vi "Protected Channel.vi"(8 "error in (no error)":errorcluster, 11 "Node Ptr":T1 format="%.0x") -> (0 "error out":errorcluster)   [LabVIEW 2015, in "Fuel Injection Addon System Explorer.lvlib"]
uses:
  Fuel Injection Addon System Explorer.lvlib
  <vilib>/NI Veristand/Custom Device API/Custom Device Item Ref.ctl
  <vilib>/NI Veristand/Custom Device API/Custom Device Channel Type.ctl
  <vilib>/NI Veristand/Custom Device API/Custom Device API.lvlib
panel:
  out "Original Name":string
  in  "Default Value":dbl
  out "Units":string
  in  "Header":cluster{"Section Name":string}={"Section Name"="Custom Device Item Settings"}
  in  "Description":string
  in  "Name":string
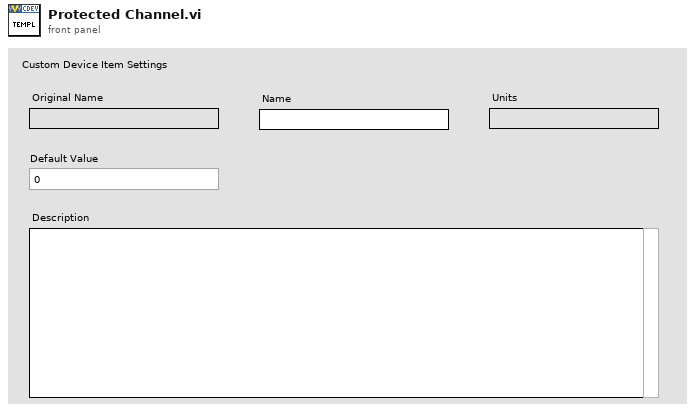
[diagram p1: front panel]
types:
  T1 = typedef "Custom Device API.lvlib/Custom Device Item Ref.ctl" = u64
  T2 = typedef "Custom Device API.lvlib/Custom Device Channel Type.ctl" = enum16{"Input", "Output"}
  T3 = typedef "Custom Device API.lvlib/Custom Device Item Info.ctl" = cluster{"Name":string, "Is Channel":bool, "GUID":string, "Is Waveform":bool}
  T4 = typedef "Custom Device API.lvlib/Custom Device Waveform.ctl" = cluster{"Data Type":T5, "Units":string}
  T5 = typedef "Custom Device API.lvlib/Custom Device Waveform DataType.ctl" = enum16{"Double", "Complex Double"}
  T6 = typedef "Custom Device API.lvlib/Custom Device Channel.ctl" = cluster{"Type":T2, "Units":string, "Default Value":dbl, "Faultable":bool, "Scalable":bool}
  T7 = typedef "Custom Device API.lvlib/Custom Device Commands.ctl" = enum16{"Default", "Item renamed", "Shutdown", "Dynamic button pressed"}
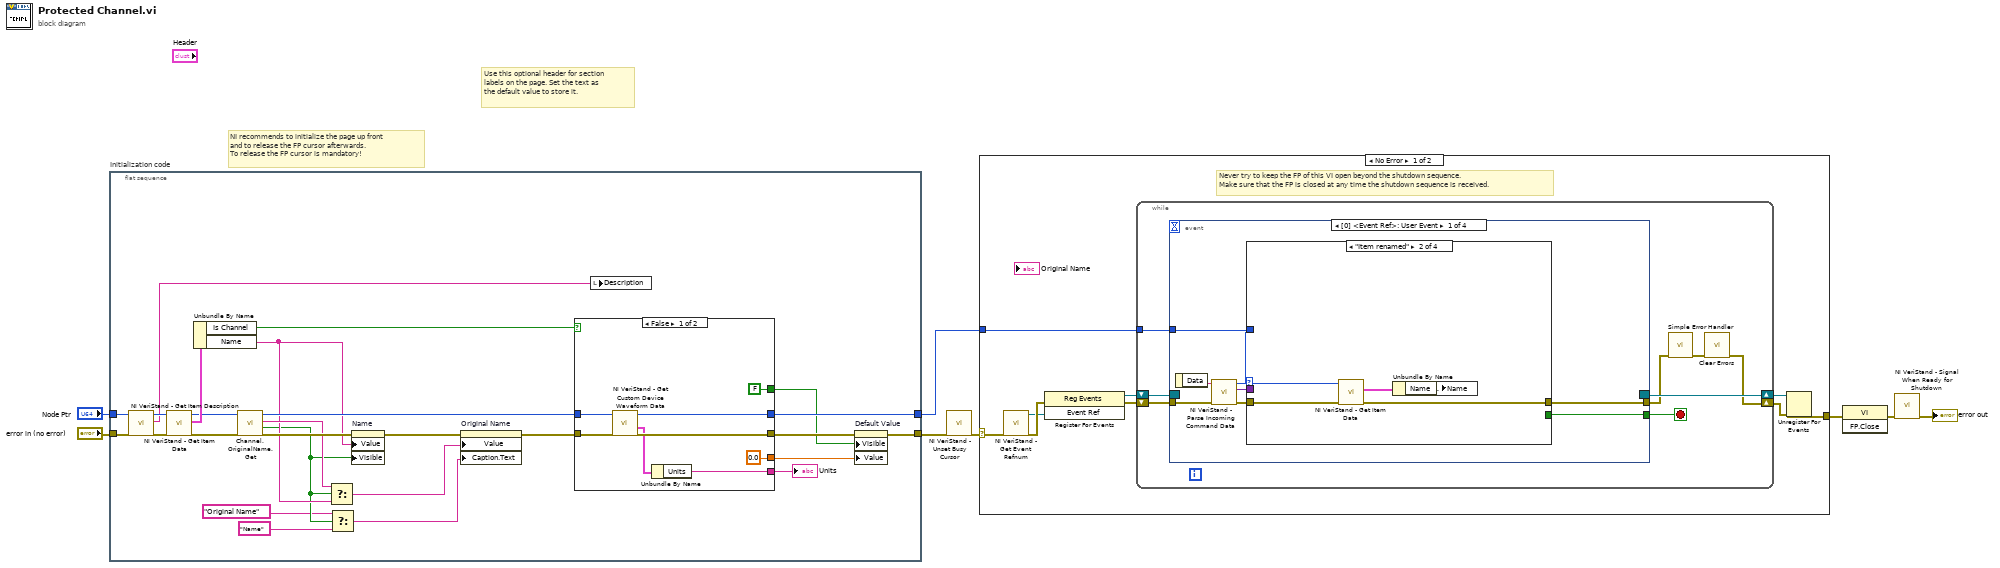
[diagram p0: block diagram]
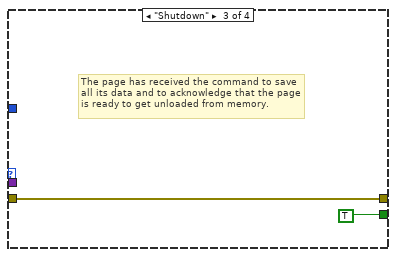
[diagram p3: hidden frame]
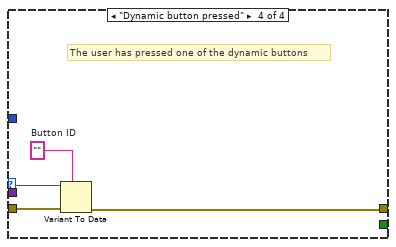
[diagram p4: hidden frame]
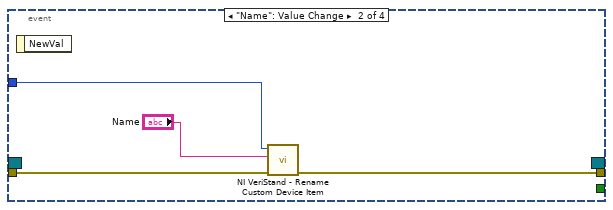
[diagram p5: hidden frame]
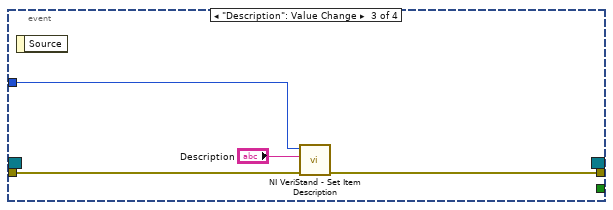
[diagram p6: hidden frame]
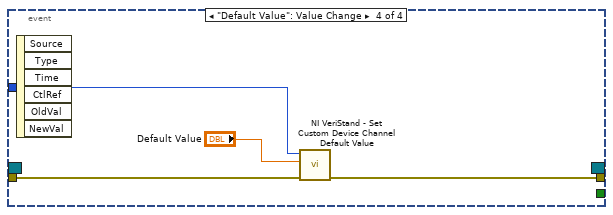
[diagram p7: hidden frame]
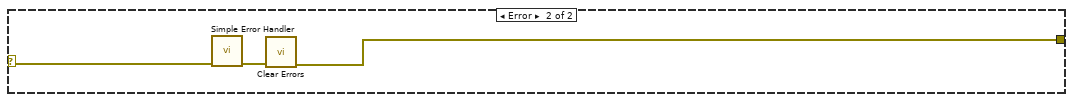
[diagram p8: hidden frame]
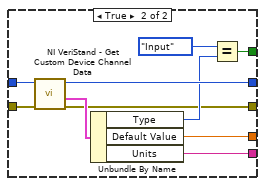
[diagram p9: hidden frame]
diagram:
  # "Use this optional header for section labels on the page. Set the text as the default value to store it."
  # "NI recommends to initialize the page up front\nand to release the FP cursor afterwards.\nTo release the FP cursor is mandatory!"
  n1 = flat-sequence "Initialization code" {
    tunnel: "error in (no error)" -> [w33]
    tunnel: "Node Ptr" -> [w32]
    tunnel: [w24] -> w4
    tunnel: [w28] -> w1
    frame #0 {
      n2 = call <vilib>:"NI VeriStand - Get Item Description.vi"("error in (no error)"=w33, "Item Ref in"=w32) -> ("error out"=w30:errorcluster, "Description"=w31:string, "Item Ref out"=w34:T1)  [unwired: 7 out]
      n3 = call <vilib>:"NI VeriStand - Get Item Data.vi"("error in (no error)"=w30, "Item Ref in"=w34) -> ("error out"=w20:errorcluster, "Item Info"=w29:T3, "Item Ref out"=w21:T1)  [unwired: 7 out]
      n4 = Unbundle By Name(w29) -> ("Is Channel"=w22:bool, "Name"=w14:string)
      n5 = call "Channel.OriginalName.Get.vi"("error in (no error)"=w20, "Ref in"=w21) -> ("error out"=w19:errorcluster, "Found?"=w12:bool, "Value"=w15:string, "Ref out"=w18:T1)  [unwired: 6 in]
      n6 = Select(t=w15, s=w12, f=w14) -> (s? t:f=w13:string)
      n7 = Select(t="Original Name" ("s? t:f"), s=w12, f="Name" ("s? t:f")) -> (s? t:f=w9:string)
      n8 = property on="Name" class="Str"(error in=w19, "Value"=w14, "Visible"=w12) -> (error out=w17:errorcluster)  [unwired: 1 in, 1 out]
      n9 = property on="Original Name" class="Str"(error in=w17, "Value"=w13, "Caption.Text"=w9) -> (error out=w16:errorcluster)  [unwired: 1 in, 1 out]
      n10 = case shown="False" w22 {
        tunnel: w18 -> [w42 w51]
        tunnel: [w39 w50] -> w28
        tunnel: w16 -> [w41 w49]
        tunnel: [w35 w48] -> w27
        tunnel: [0.0 ("Default Value") w45] -> w26
        tunnel: [w40 w44] -> w25
        tunnel: [FALSE w43] -> w23
        frame False {
          n11 = call <vilib>:"NI VeriStand - Get Custom Device Waveform Data.vi"("error in (no error)"=w41, "Waveform Ref in"=w42) -> ("error out"=w40:errorcluster, "Waveform"=w36:T4, "Waveform Ref out"=w39:T1)  [unwired: 4 in, 3 out]
          n12 = Unbundle By Name(w36) -> ("Units"=w35:string)
        }
        frame True {
          n13 = call <vilib>:"NI VeriStand - Get Custom Device Channel Data.vi"("error in (no error)"=w49, "Channel Ref in"=w51) -> ("error out"=w44:errorcluster, "Channel"=w52:T6, "Channel Ref out"=w50:T1)  [unwired: 4 in, 3 out]
          n14 = Unbundle By Name(w52) -> ("Type"=w47:T2, "Default Value"=w45:dbl, "Units"=w48:string)
          n15 = Equal?(x=Custom_Device_Channel_Type."Input", y=w47) -> (x = y?=w43:bool)
        }
      }
      "Units" <- w27
      n16 = local write "Description"(w31) -> ()
      n17 = property on="Default Value" class="DigNum (strict)"(error in=w25, "Visible"=w23, "Value"=w26) -> (error out=w24:errorcluster)  [unwired: 1 in, 1 out]
    }
  }
  n18 = call <vilib>:"NI VeriStand - Unset Busy Cursor.vi"("error in (no error)"=w4) -> ("error out"=w3:errorcluster)  [unwired: 10 out]
  n19 = case shown="No Error" w3 {
    selector: w3 -> [w53 w104]
    tunnel: [w58 w102] -> w8
    tunnel: w1 -> [w54 _]
    frame No Error {
      # "Never try to keep the FP of this VI open beyond the shutdown sequence.\nMake sure that the FP is closed at any time the shutdown sequence is received."
      n20 = call <vilib>:"NI VeriStand - Get Event Refnum.vi"("error in (no error)"=w53) -> ("error out"=w61:errorcluster, "Event Ref"=w57:refnum<user-event>)  [unwired: 9 out]
      n21 = register-events(error in=w61, w57) -> (reference out=w55:refnum<event-registration>, error out=w56:errorcluster)  [unwired: 1 in]
      n22 = while {
        tunnel: w54 -> [w65]
        shift-right: [w62] -> w59
        shift-left: w56 -> [w68]
        shift-right: [w69] -> w60
        shift-left: w55 -> [w67]
        stop <- w66 stop-if-true
        n23 = event shown="[0] <Event Ref>: User Event" {
          selector: w67 -> [_ _ _ _]
          dyn-events: [_ _ _ _] -> w69
          timeout: _ -> [_ _ _ _]
          tunnel: w68 -> [w77 w93 w96 w100]
          tunnel: [w73 _ _ _] -> w66
          tunnel: [w72 w92 w95 w99] -> w64
          tunnel: w65 -> [w71 w91 w97 w101]
          event User Event {
            n24 = event-data() -> ("Data"=w76:string)  [unwired: 1 out]
            n25 = call <vilib>:"NI VeriStand - Parse Incoming Command Data.vi"("error in (no error)"=w77, "Incoming data"=w76) -> ("error out"=w75:errorcluster, "Outgoing data"=w70:variant, "Action"=w74:T7)  [unwired: 7 out]
            n26 = case shown="\"Item renamed\"" w74 {
              tunnel: w75 -> [w78 w83 w84 w89]
              tunnel: [_ _ TRUE _] -> w73
              tunnel: [w78 w80 w84 w86] -> w72
              tunnel: w71 -> [_ w82 _ _]
              tunnel: w70 -> [_ _ _ w88]
              frame "Default", Default {
              }
              frame "Item renamed" {
                n27 = call <vilib>:"NI VeriStand - Get Item Data.vi"("error in (no error)"=w83, "Item Ref in"=w82) -> ("error out"=w80:errorcluster, "Item Info"=w81:T3)  [unwired: 8 out]
                n28 = Unbundle By Name(w81) -> ("Name"=w79:string)
                n29 = local write "Name"(w79) -> ()
              }
              frame "Shutdown" {
                # "The page has received the command to save all its data and to acknowledge that the page is ready to get unloaded from memory."
              }
              frame "Dynamic button pressed" {
                w87 = ""  # Button ID
                # "The user has pressed one of the dynamic buttons"
                n30 = Variant To Data(error in=w89, type=w87, Variant=w88) -> (error out=w86:errorcluster)  [unwired: 1 out]
              }
            }
          }
          event "Name": Value Change {
            n31 = event-data() -> ()  [unwired: 2 out]
            n32 = call <vilib>:"NI VeriStand - Rename Custom Device Item.vi"("error in (no error)"=w93, "New Name"="Name", "Item Ref in"=w91) -> ("error out"=w92:errorcluster)  [unwired: 1 in, 7 out]
          }
          event "Description": Value Change {
            n33 = event-data() -> ()  [unwired: 2 out]
            n34 = call <vilib>:"NI VeriStand - Set Item Description.vi"("error in (no error)"=w96, "Description"="Description", "Item Ref in"=w97) -> ("error out"=w95:errorcluster)  [unwired: 8 out]
          }
          event "Default Value": Value Change {
            n35 = event-data() -> ()  [unwired: 7 out]
            n36 = call <vilib>:"NI VeriStand - Set Custom Device Channel Default Value.vi"("error in (no error)"=w100, "Default Value"="Default Value", "Channel Ref in"=w101) -> ("error out"=w99:errorcluster)  [unwired: 7 in, 1 out]
          }
        }
        n37 = call <vilib>:"Simple Error Handler.vi"("error in (no error)"=w64) -> ("error out"=w63:errorcluster)  [unwired: 1 in, 7 out]
        n38 = call <vilib>:"Clear Errors.vi"("error in (no error)"=w63) -> ("error out"=w62:errorcluster)  [unwired: 1 in, 5 out]
      }
      n39 = Unregister For Events(event registration refnum=w60, error in=w59) -> (error out=w58:errorcluster)
    }
    frame Error {
      n40 = call <vilib>:"Simple Error Handler.vi"("error in (no error)"=w104) -> ("error out"=w103:errorcluster)  [unwired: 1 in, 7 out]
      n41 = call <vilib>:"Clear Errors.vi"("error in (no error)"=w103) -> ("error out"=w102:errorcluster)  [unwired: 1 in, 5 out]
    }
  }
  n42 = invoke class="VI" method="FP.Close"(error in=w8) -> (error out=w7:errorcluster)  [unwired: 2 in, 2 out]
  n43 = call <vilib>:"NI VeriStand - Signal When Ready for Shutdown.vi"("error in (no error)"=w7) -> ("error out"=→"error out":errorcluster)  [unwired: 10 out]
